vi "VI Tree.vi"   [LabVIEW 2011, in "Thorlabs_MDT69xB.lvlib"]
doc: "This is the instrument driver for the <INSTRUMENT NAME>. The VI Tree displays all the user-callable VIs of the instrument driver in an organized table."
uses:
  <instrlib>/Thorlabs_MDT69xB/Thorlabs_MDT69xB.lvlib
panel:
  # "(c) 2009 <Enter Company Name Here>.  ALL RIGHTS RESERVED."
  # "SEE DIAGRAM\nFOR VI TREE."
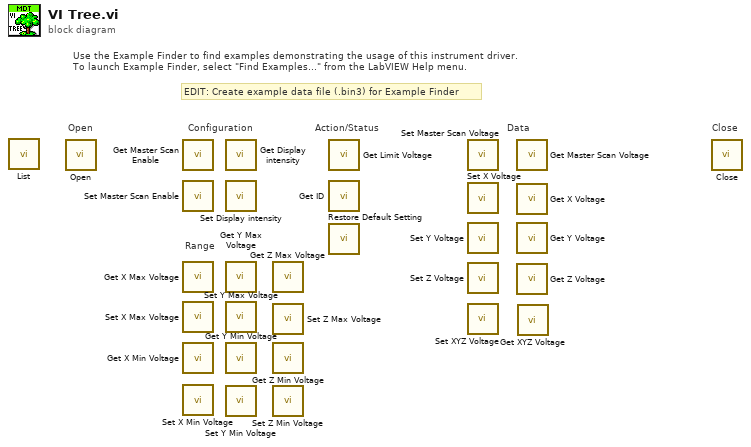
[diagram p0: block diagram]
diagram:
  # "Range"
  # "Open"
  # "EDIT: Create example data file (.bin3) for Example Finder"
  # "Use the Example Finder to find examples demonstrating the usage of this instrument driver.\nTo launch Example Finder, select \"Find Examples...\" from the LabVIEW Help menu."
  # "Configuration"
  # "Data"
  # "Action/Status"
  # "Close"
  n1 = call <instrlib>:"List.vi"() -> ()  [unwired: 10 in, 2 out]
  n2 = call <instrlib>:"Open.vi"() -> ()  [unwired: 9 in, 3 out]
  n3 = call <instrlib>:"Get Master Scan Enable.vi"() -> ()  [unwired: 9 in, 3 out]
  n4 = call <instrlib>:"Set Master Scan Enable.vi"() -> ()  [unwired: 10 in, 2 out]
  n5 = call <instrlib>:"Get X Max Voltage.vi"() -> ()  [unwired: 9 in, 3 out]
  n6 = call <instrlib>:"Set X Max Voltage.vi"() -> ()  [unwired: 10 in, 2 out]
  n7 = call <instrlib>:"Get X Min Voltage.vi"() -> ()  [unwired: 9 in, 3 out]
  n8 = call <instrlib>:"Set X Min Voltage.vi"() -> ()  [unwired: 10 in, 2 out]
  n9 = call <instrlib>:"Get Display intensity.vi"() -> ()  [unwired: 9 in, 3 out]
  n10 = call <instrlib>:"Set Display intensity.vi"() -> ()  [unwired: 10 in, 2 out]
  n11 = call <instrlib>:"Get Y Max Voltage.vi"() -> ()  [unwired: 9 in, 3 out]
  n12 = call <instrlib>:"Set Y Max Voltage.vi"() -> ()  [unwired: 10 in, 2 out]
  n13 = call <instrlib>:"Get Y Min Voltage.vi"() -> ()  [unwired: 9 in, 3 out]
  n14 = call <instrlib>:"Set Y Min Voltage.vi"() -> ()  [unwired: 10 in, 2 out]
  n15 = call <instrlib>:"Get Z Max Voltage.vi"() -> ()  [unwired: 9 in, 3 out]
  n16 = call <instrlib>:"Set Z Max Voltage.vi"() -> ()  [unwired: 10 in, 2 out]
  n17 = call <instrlib>:"Get Z Min Voltage.vi"() -> ()  [unwired: 9 in, 3 out]
  n18 = call <instrlib>:"Set Z Min Voltage.vi"() -> ()  [unwired: 10 in, 2 out]
  n19 = call <instrlib>:"Get Limit Voltage.vi"() -> ()  [unwired: 9 in, 3 out]
  n20 = call <instrlib>:"Get ID.vi"() -> ()  [unwired: 9 in, 3 out]
  n21 = call <instrlib>:"Restore Default Setting.vi"() -> ()  [unwired: 10 in, 2 out]
  n22 = call <instrlib>:"Set Master Scan Voltage.vi"() -> ()  [unwired: 10 in, 2 out]
  n23 = call <instrlib>:"Set X Voltage.vi"() -> ()  [unwired: 10 in, 2 out]
  n24 = call <instrlib>:"Set Y Voltage.vi"() -> ()  [unwired: 10 in, 2 out]
  n25 = call <instrlib>:"Set Z Voltage.vi"() -> ()  [unwired: 10 in, 2 out]
  n26 = call <instrlib>:"Set XYZ Voltage.vi"() -> ()  [unwired: 10 in, 2 out]
  n27 = call <instrlib>:"Get Master Scan Voltage.vi"() -> ()  [unwired: 9 in, 3 out]
  n28 = call <instrlib>:"Get X Voltage.vi"() -> ()  [unwired: 9 in, 3 out]
  n29 = call <instrlib>:"Get Y Voltage.vi"() -> ()  [unwired: 9 in, 3 out]
  n30 = call <instrlib>:"Get Z Voltage.vi"() -> ()  [unwired: 9 in, 3 out]
  n31 = call <instrlib>:"Get XYZ Voltage.vi"() -> ()  [unwired: 7 in, 5 out]
  n32 = call <instrlib>:"Close.vi"() -> ()  [unwired: 11 in, 1 out]
